vi "executeQuery.vi"(8 "error in (no error)":errorcluster, 10 "command":string, 11 "AlCS in":refnum<class "AlCS.lvclass">) -> (0 "error out":errorcluster, 2 "answer":string, 3 "AlCS out":refnum<class "AlCS.lvclass">)   [LabVIEW 2016, in "AlCS.lvclass"]
uses:
  AlCS.lvclass
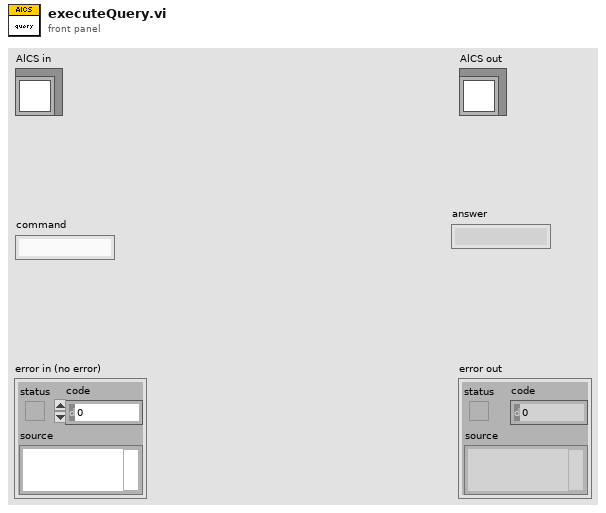
[diagram p1: front panel]
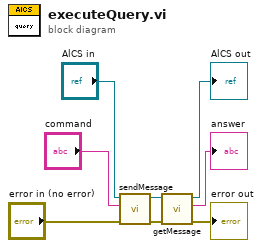
[diagram p0: block diagram]
diagram:
  n1 = call "sendMessage.vi"("error in (no error)"="error in (no error)", "message"="command", "AlCS in"="AlCS in") -> ("error out"=w8:errorcluster, "AlCS out"=w7:refnum<class "AlCS.lvclass">)  [unwired: 7 in]
  n2 = call "getMessage.vi"("error in (no error)"=w8, "AlCS in"=w7) -> ("error out"=→"error out":errorcluster, "message"=→"answer":string, "AlCS out"=→"AlCS out":refnum<class "AlCS.lvclass">)  [unwired: 7 in]
